vi "Send Message.vi"(8 "error in (no error)":errorcluster, 10 "Message":string, 11 "Channel GUI in":refnum<class "Channel GUI.lvclass">) -> (0 "error out":errorcluster, 3 "Channel GUI out":refnum<class "Channel GUI.lvclass">)   [LabVIEW 2018, in "Channel GUI.lvclass"]
uses:
  Channel GUI.lvclass
  Channel GUI.lvclass/Channel GUI.ctl
  Stream/Stream.lvclass
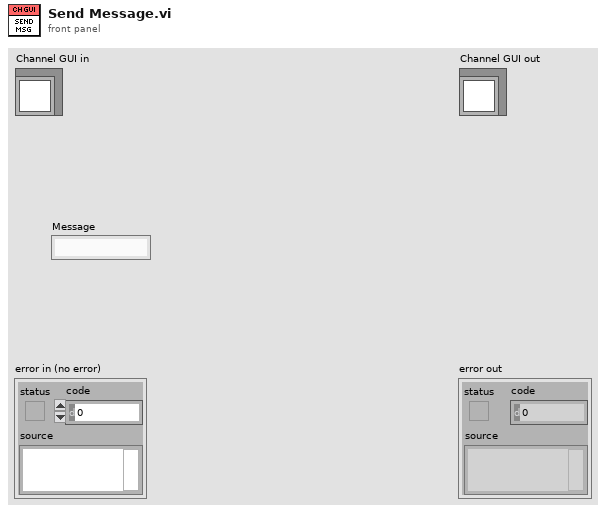
[diagram p1: front panel]
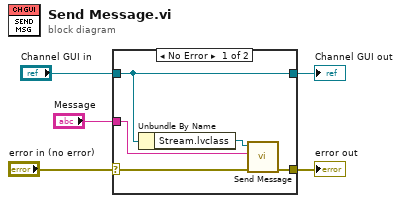
[diagram p0: block diagram]
diagram:
  n1 = case shown="No Error" "error in (no error)" {
    selector: "error in (no error)" -> [w8 w12]
    tunnel: [w7 w12] -> w4
    tunnel: [w10 w11] -> w2
    tunnel: "Channel GUI in" -> [w10 w11]
    tunnel: "Message" -> [w6 _]
    frame No Error {
      n2 = Unbundle By Name(w10) -> ("Stream.lvclass"=w9:refnum<class "Stream.lvclass">)
      n3 = call "Send Message.vi"("error in (no error)"=w8, "Message"=w6, "Stream in"=w9) -> ("error out"=w7:errorcluster)  [unwired: 7 in, 1 out]
    }
    frame Error {
    }
  }
  "error out" <- w4
  "Channel GUI out" <- w2
